vi "tcp server testing.vi"() -> ()   [LabVIEW 2015]
uses:
  connection/connection maintainer.lvclass
  message/communicator message.lvclass
  communicator/communicator.lvclass/communicator.ctl
  TCP/TCP server.lvclass
  communicator/communicator.lvclass
panel:
  out "data 4":variant
  out "ID 4":string
  out "data 3":variant
  out "ID 3":string
  in  "stop 2":bool
  out "queue":refnum<class "connection maintainer.lvclass">
  out "error out 4":errorcluster
  out "error out 3":errorcluster
  out "error out 2":errorcluster
  out "error out":errorcluster
  in  "tcp":bool
  in  "data 2":string
  in  "ID 2":string
  in  "data":string
  in  "ID":string
  in  "stop":bool
  in  "send":bool
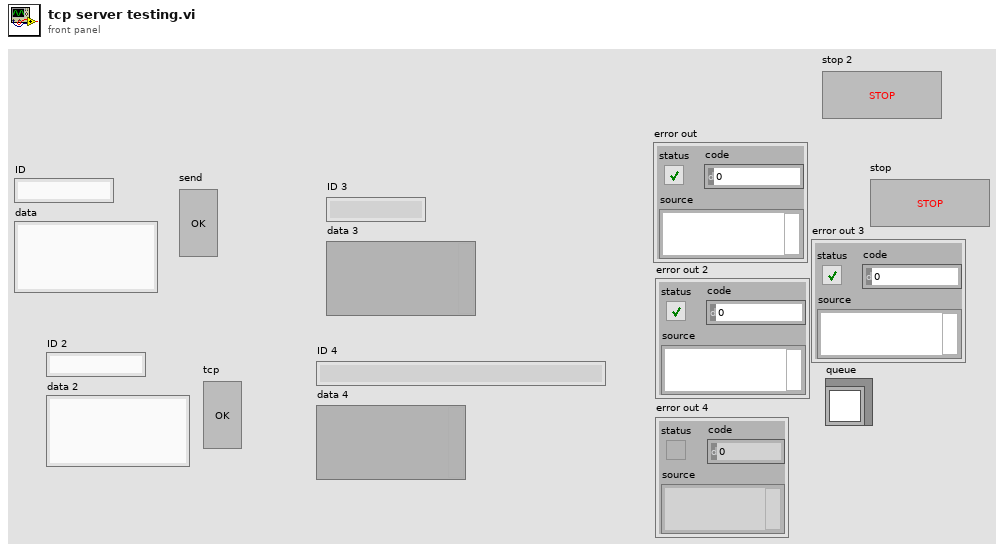
[diagram p1: front panel]
types:
  T1 = enum16{"Standard", "Buffered", "CRLF", "Immediate"}
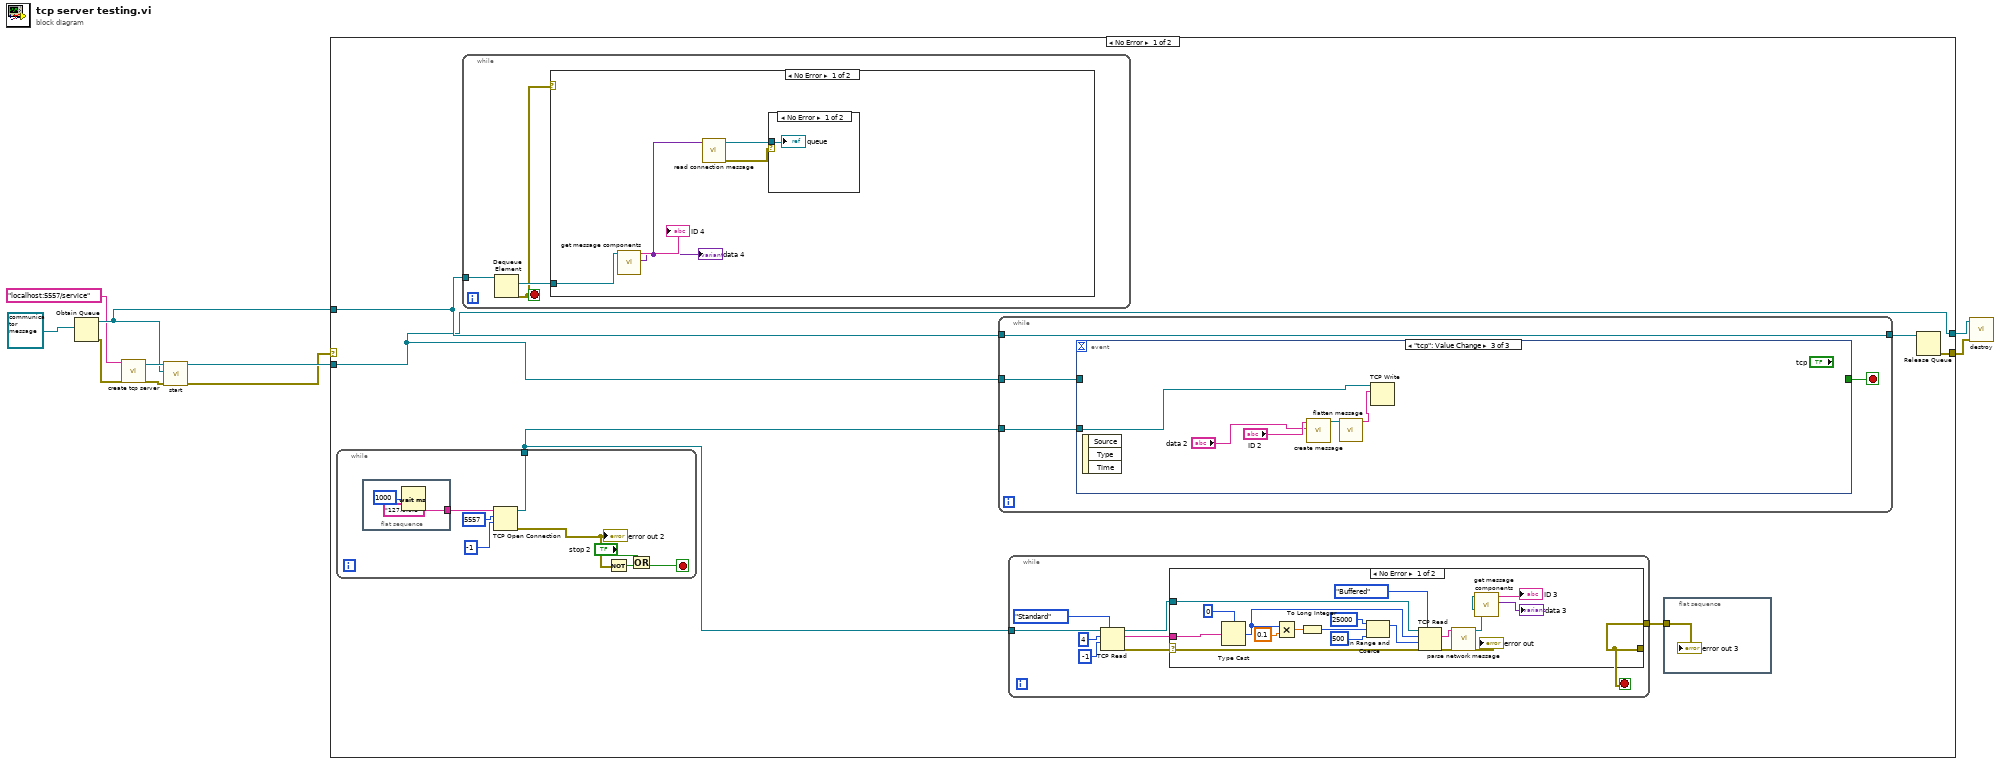
[diagram p0: block diagram]
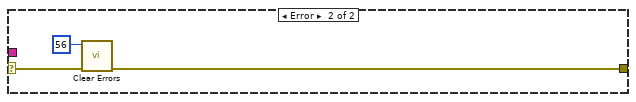
[diagram p2: hidden frame]
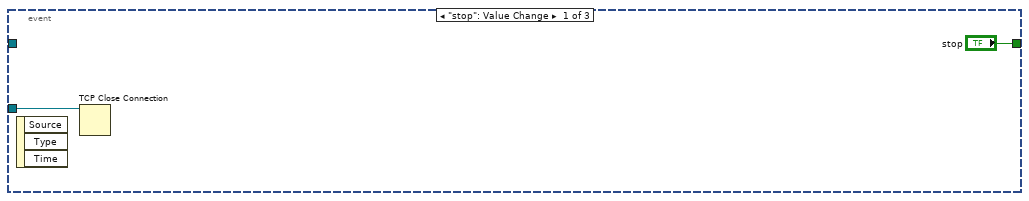
[diagram p3: hidden frame]
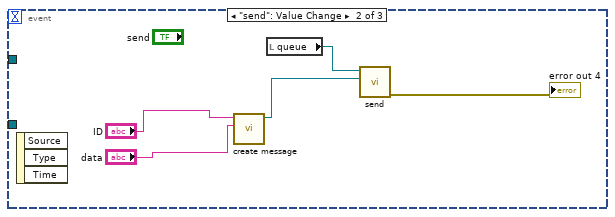
[diagram p4: hidden frame]
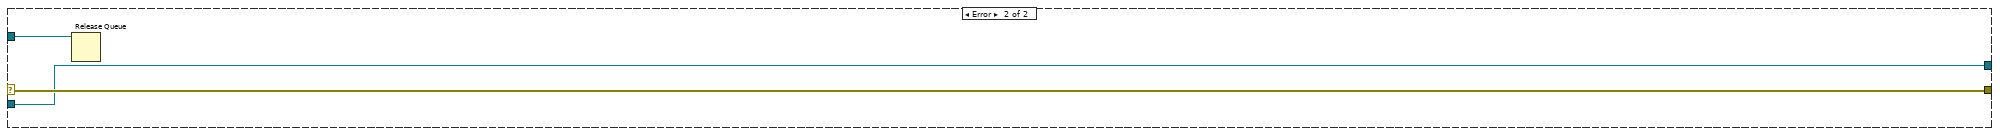
[diagram p7: hidden frame]
diagram:
  n1 = Obtain Queue(element data type=refnum<class "communicator message.lvclass"> refnum ("message")) -> (queue out=w6:refnum<queue>, error out=w2:errorcluster)  [unwired: 4 in, 1 out]
  n2 = call "create tcp server.vi"("error in"=w2, "conn string"="localhost:5557/service" ("connection string")) -> ("error out"=w7:errorcluster, "TCP server out"=w8:refnum<class "TCP server.lvclass">)  [unwired: 8 in]
  n3 = call-dynamic "start.vi"("error in"=w7, "queue to parent"=w6, "communicator in"=w8) -> ("error out"=w3:errorcluster, "communicator out"=w4:refnum<class "TCP server.lvclass">)  [unwired: 7 in]
  n4 = case shown="No Error" w3 {
    selector: w3 -> [_ w84]
    tunnel: [w11 w82] -> w10
    tunnel: w6 -> [w16 w83]
    tunnel: [w14 w84] -> w9
    tunnel: w4 -> [w11 w82]
    frame No Error {
      n5 = while {
        tunnel: [w22] -> w13
        stop <- w19 stop-if-true
        n6 = flat-sequence {
          tunnel: ["127.0.0.1" ("address")] -> w24
          frame #0 {
            n7 = Wait (ms)(milliseconds to wait=u32 1000) -> ()  [unwired: 1 out]
          }
        }
        n8 = TCP Open Connection(address=w24, remote port or service name=u16 5557, timeout ms (60000)=-1) -> (connection ID=w22:refnum<k5>, error out=w20:errorcluster)  [unwired: 2 in]
        "error out 2" <- w20
        n9 = Not(x=w20) -> (.not. x?=w17:bool)
        n10 = Or(x="stop 2", y=w17) -> (x .or. y?=w19:bool)
      }
      n11 = while {
        tunnel: w16 -> [w75]
        stop <- w73 stop-if-true
        n12 = Dequeue Element(queue=w75) -> (element=w74:refnum<class "communicator message.lvclass">, error out=w73:errorcluster)  [unwired: 2 in, 2 out]
        n13 = case shown="No Error" w73 {
          tunnel: w74 -> [w77 _]
          frame No Error {
            n14 = call "get message components.vi"("message"=w77) -> ("data"=w76:variant, "ID"=→"ID 4":string)  [unwired: 9 in]
            "data 4" <- w76
            n15 = call "read connection message.vi"("data"=w76) -> ("error out"=w79:errorcluster, "conn"=w80:refnum<class "connection maintainer.lvclass">)  [unwired: 9 in]
            n16 = case shown="No Error" w79 {
              tunnel: w80 -> [w81 _]
              frame No Error {
                "queue" <- w81
              }
              frame Error {
              }
            }
          }
          frame Error {
          }
        }
      }
      n17 = while {
        tunnel: w11 -> [w58]
        tunnel: [w59] -> w15
        tunnel: w16 -> [w59]
        tunnel: w13 -> [w57]
        stop <- w60 stop-if-true
        n18 = event shown="[2] \"tcp\": Value Change" {
          selector: _ -> [_ _ _]
          dyn-events: _ -> [_ _ _]
          timeout: _ -> [_ _ _]
          tunnel: ["stop" _ _] -> w60
          tunnel: w58 -> [_ _ _]
          tunnel: w57 -> [w61 _ w71]
          event "stop": Value Change {
            n19 = event-data() -> ()  [unwired: 1 in, 3 out]
            n20 = TCP Close Connection(connection ID=w61) -> ()  [unwired: 2 in, 2 out]
          }
          event "send": Value Change {
            n21 = event-data() -> ()  [unwired: 1 in, 3 out]
            n22 = call "create message.vi"("data"="data", "ID"="ID") -> ("message"=w63:refnum<class "communicator message.lvclass">)  [unwired: 9 in]
            n23 = local read "queue"() -> (w67:refnum<class "connection maintainer.lvclass">)
            n24 = call "send.vi"("element"=w63, "communicator in"=w67) -> ("error out"=→"error out 4":errorcluster)  [unwired: 9 in]
          }
          event "tcp": Value Change {
            n25 = event-data() -> ()  [unwired: 1 in, 3 out]
            n26 = call "create message.vi"("data"="data 2", "ID"="ID 2") -> ("message"=w70:refnum<class "communicator message.lvclass">)  [unwired: 9 in]
            n27 = call "flatten message.vi"("data message"=w70) -> ("data"=w72:string)  [unwired: 9 in, 1 out]
            n28 = TCP Write(connection ID=w71, data in=w72) -> ()  [unwired: 2 in, 3 out]
          }
        }
      }
      n29 = while {
        tunnel: w13 -> [w29]
        tunnel: [w28] -> w12
        stop <- w28 stop-if-true
        n30 = TCP Read(connection ID=w29, bytes to read=4, 7:T1."Standard" ("mode (standard)"), 9:-1 ("timeout ms (25000)")) -> (connection ID out=w35:refnum<k5>, data out=w34:string, error out=w33:errorcluster)  [unwired: 1 in]
        n31 = case shown="No Error" w33 {
          selector: w33 -> [w50 w56]
          tunnel: [_ w54] -> w28
          tunnel: w34 -> [w53 _]
          tunnel: w35 -> [w51 _]
          frame No Error {
            n32 = Type Cast(type=0, x=w53) -> (*(type *) &x=w45:i32)
            n33 = Multiply(x=w45, y=0.1) -> (x*y=w46:dbl)
            n34 = To Long Integer(number=w46) -> (32bit integer=w41:i32)
            n35 = In Range and Coerce(upper limit=25000 ("timeout ms (25000)"), x=w41, lower limit=500 ("timeout ms (25000)")) -> (coerced(x)=w42:i32)  [unwired: 1 out]
            n36 = TCP Read(connection ID=w51, bytes to read=w45, error in (no error)=w50, 7:T1."Buffered" ("mode (standard)"), 9:w42) -> (data out=w49:string, error out=w40:errorcluster)  [unwired: 1 out]
            n37 = call "parse network message.vi"("error in"=w40, "data"=w49) -> ("error out"=→"error out":errorcluster, "message"=w37:refnum<class "communicator message.lvclass">)  [unwired: 8 in]
            n38 = call "get message components.vi"("message"=w37) -> ("data"=→"data 3":variant, "ID"=→"ID 3":string)  [unwired: 9 in]
          }
          frame Error {
            n39 = call <vilib>:"Clear Errors.vi"("error in (no error)"=w56, "specific error code to clear (0: all)"=56) -> ("error out"=w54:errorcluster)  [unwired: 4 in, 1 out]
          }
        }
      }
      n40 = flat-sequence {
        tunnel: w12 -> [w27]
        frame #0 {
          "error out 3" <- w27
        }
      }
      n41 = Release Queue(queue=w15) -> (error out=w14:errorcluster)  [unwired: 2 in, 2 out]
    }
    frame Error {
      n42 = Release Queue(queue=w83) -> ()  [unwired: 2 in, 3 out]
    }
  }
  n43 = call-dynamic "destroy.vi"("error in"=w9, "communicator in"=w10) -> ()  [unwired: 9 in, 1 out]
